vi "problem2.vi"() -> ()   [LabVIEW 2022 SP3]
uses:
  7b43adb1-cacc-2e4f-b1ac-163facdfa357.vi
panel:
  in  "Play":bool
  out "Bank":dbl
  in  "stop":bool
  in  "user array":i32[](array[numeric])
  out "Final value":i32
  in  "Bet Amount":i32
  out "output array 2":i32[](array[numeric])
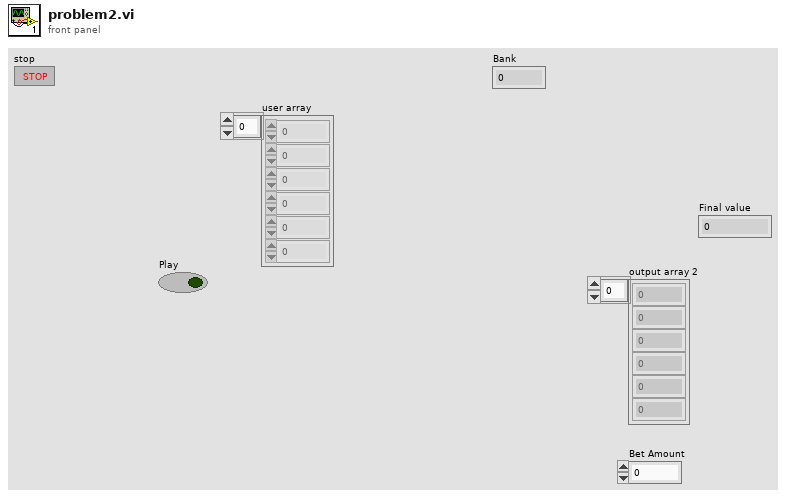
[diagram p1: front panel]
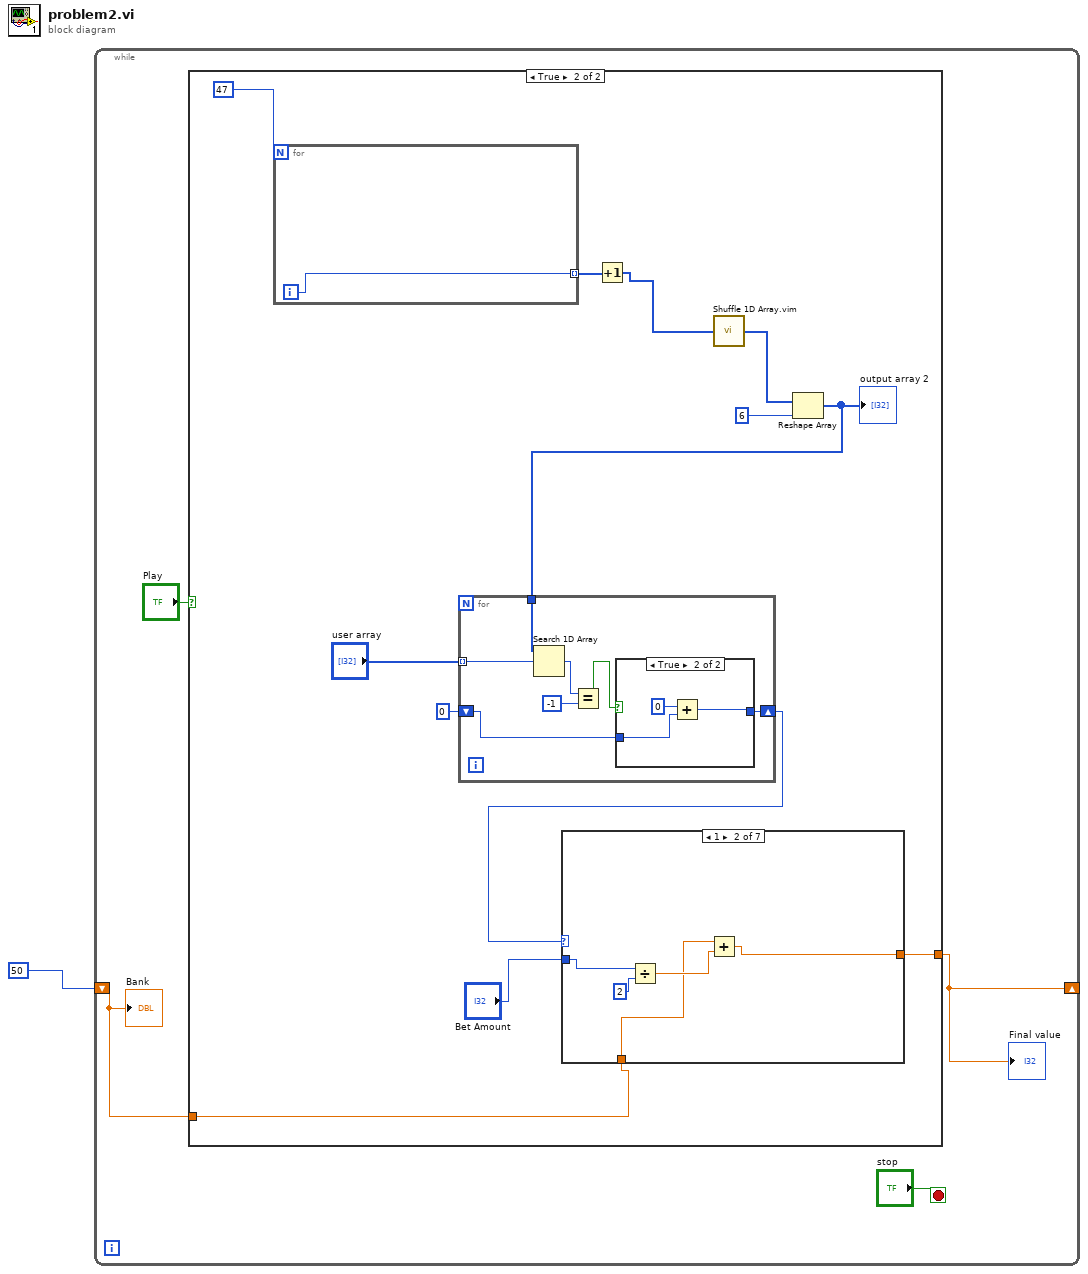
[diagram p0: block diagram]
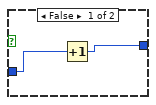
[diagram p3: hidden frame]
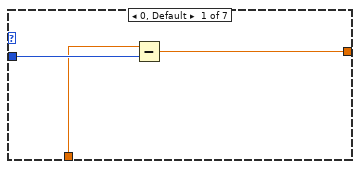
[diagram p4: hidden frame]
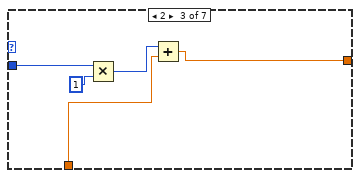
[diagram p5: hidden frame]
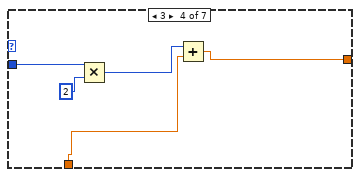
[diagram p6: hidden frame]
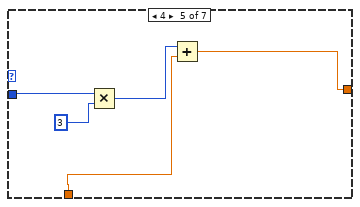
[diagram p7: hidden frame]
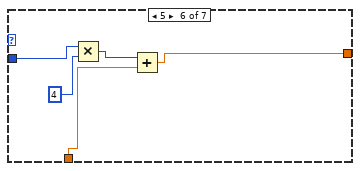
[diagram p8: hidden frame]
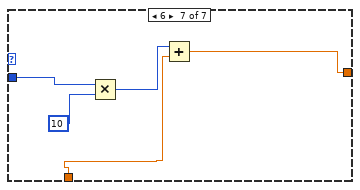
[diagram p9: hidden frame]
diagram:
  n1 = while {
    shift-right: [w2] -> _
    shift-left: 50 ("Bank") -> [w5]
    stop <- "stop" stop-if-true
    n2 = case shown="True" "Play" {
      tunnel: w5 -> [w6 w12]
      tunnel: [w6 w11] -> w2
      frame False {
      }
      frame True {
        n3 = for {
          N: 47 -> [_]
          tunnel: [w64] -> w17 mode=indexing
          i -> [w64]
        }
        n4 = Increment(x=w17) -> (x+1=w16:i32[])
        n5 = call "Shuffle 1D Array.vim"("array"=w16) -> ("shuffled array"=w14:i32[])  [unwired: 4 in]
        n6 = Reshape Array(w14, 6) -> (w10:i32[])
        "output array 2" <- w10
        n7 = for {
          tunnel: w10 -> [w25]
          tunnel: "user array" -> [w24] mode=indexing
          shift-right: [w20] -> w8
          shift-left: 0 -> [w19]
          n8 = Search 1D Array(1D array=w25, element=w24) -> (index of element=w23:i32)  [unwired: 1 in]
          n9 = Equal?(x=w23, y=-1) -> (x = y?=w22:bool)
          n10 = case shown="True" w22 {
            tunnel: [w26 w28] -> w20
            tunnel: w19 -> [w27 w29]
            frame False {
              n11 = Increment(x=w27) -> (x+1=w26:i32)
            }
            frame True {
              n12 = Add(x=0, y=w29) -> (x+y=w28:i32)
            }
          }
        }
        n13 = case shown="1" w8 {
          tunnel: "Bet Amount" -> [w33 w38 w43 w48 w53 w58 w63]
          tunnel: w12 -> [w32 w35 w40 w45 w50 w55 w60]
          tunnel: [w31 w34 w39 w44 w49 w54 w59] -> w11
          frame 0, Default {
            n14 = Subtract(x=w32, y=w33) -> (x-y=w31:dbl)
          }
          frame 1 {
            n15 = Divide(x=w38, y=2) -> (x/y=w36:dbl)
            n16 = Add(x=w35, y=w36) -> (x+y=w34:dbl)
          }
          frame 2 {
            n17 = Multiply(x=w43, y=1) -> (x*y=w41:i32)
            n18 = Add(x=w41, y=w40) -> (x+y=w39:dbl)
          }
          frame 3 {
            n19 = Multiply(x=w48, y=2) -> (x*y=w46:i32)
            n20 = Add(x=w46, y=w45) -> (x+y=w44:dbl)
          }
          frame 4 {
            n21 = Multiply(x=w53, y=3) -> (x*y=w51:i32)
            n22 = Add(x=w51, y=w50) -> (x+y=w49:dbl)
          }
          frame 5 {
            n23 = Multiply(x=w58, y=4) -> (x*y=w56:i32)
            n24 = Add(x=w56, y=w55) -> (x+y=w54:dbl)
          }
          frame 6 {
            n25 = Multiply(x=w63, y=10) -> (x*y=w61:i32)
            n26 = Add(x=w61, y=w60) -> (x+y=w59:dbl)
          }
        }
      }
    }
    "Final value" <- w2
    "Bank" <- w5
  }
